vi "ARN Protokollkopf.vi"() -> (0 "Angehängtes Array":T1[][](array[typedef]), 3 "Kopfzeile":string[](array[string]))   [LabVIEW 2020, in "EPA 1065.lvlib" / "ARN Test 1065-305.lvlib"]
uses:
  ARN Test 1065-305.lvlib
  Visualisierungs Elemente/String - Ausgabefeld.ctl
  Seiten/FT-IR/FGV FT-IR Gasliste Aktionen.ctl
  Aktion FGV ARN Daten.ctl
  Sprachverwaltung/FGV Aktion Tabelle zerlegen.ctl
  Seiten/FT-IR/FT-IR.lvlib
  Sprachverwaltung/Sprachverwaltung.lvlib
  Seiten/System Einstellungen V2/System Einstellungen V2.lvlib
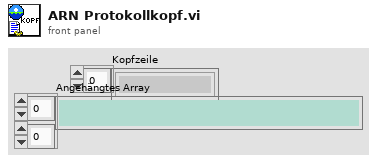
[diagram p1: front panel]
types:
  T1 = typedef "String - Ausgabefeld.ctl" = string
  T2 = typedef "Sprachverwaltung.lvlib/FGV Aktion Tabelle zerlegen.ctl" = enum16{"laden", "vereinzeln", "speichern"}
  T3 = typedef "FT-IR.lvlib/FGV FT-IR Gasliste Aktionen.ctl" = enum16{"lesen", "Gasliste FT-IR", "Gasliste ausgelesen", "laden", "speichern", "löschen"}
  T4 = typedef "EPA 1065.lvlib/ARN Test 1065-305.lvlib/Aktion FGV ARN Daten.ctl" = enum16{"Lesen", "laden", "speichern", "ARN Daten", "Rohdaten", "Rohdaten löschen", "Zeitstempel", "SNR Ergebnis"}
  T5 = typedef "EPA 1065.lvlib/ARN Test 1065-305.lvlib/Allgemeine Einstellungen.ctl" = cluster{"Bearbeiter:":string, "Analysator":T6, "Komponente:":u16, "Gasflaschen Nr.:":string, "Accuracy":dbl, "Sollwert":dbl, "Modus":T7, "Pfad:":path, "Textname:":string, "CG Aufschaltzeit:":dbl, "Einheit":string, "N2 Aufschaltzeit:":dbl, "Gasflasche":T8, "Konfig Gasflasche":T9}
  T6 = typedef "System Einstellungen V2.lvlib/Analysatoren.ctl" = string
  T7 = typedef "EPA 1065.lvlib/T90 Test 1065-308.lvlib/Modus.ctl" = u16
  T8 = typedef "System Einstellungen V2.lvlib/Gasflasche Auswahl.ctl" = u16
  T9 = typedef "System Einstellungen V2.lvlib/Konfig Gasflasche.ctl" = bool
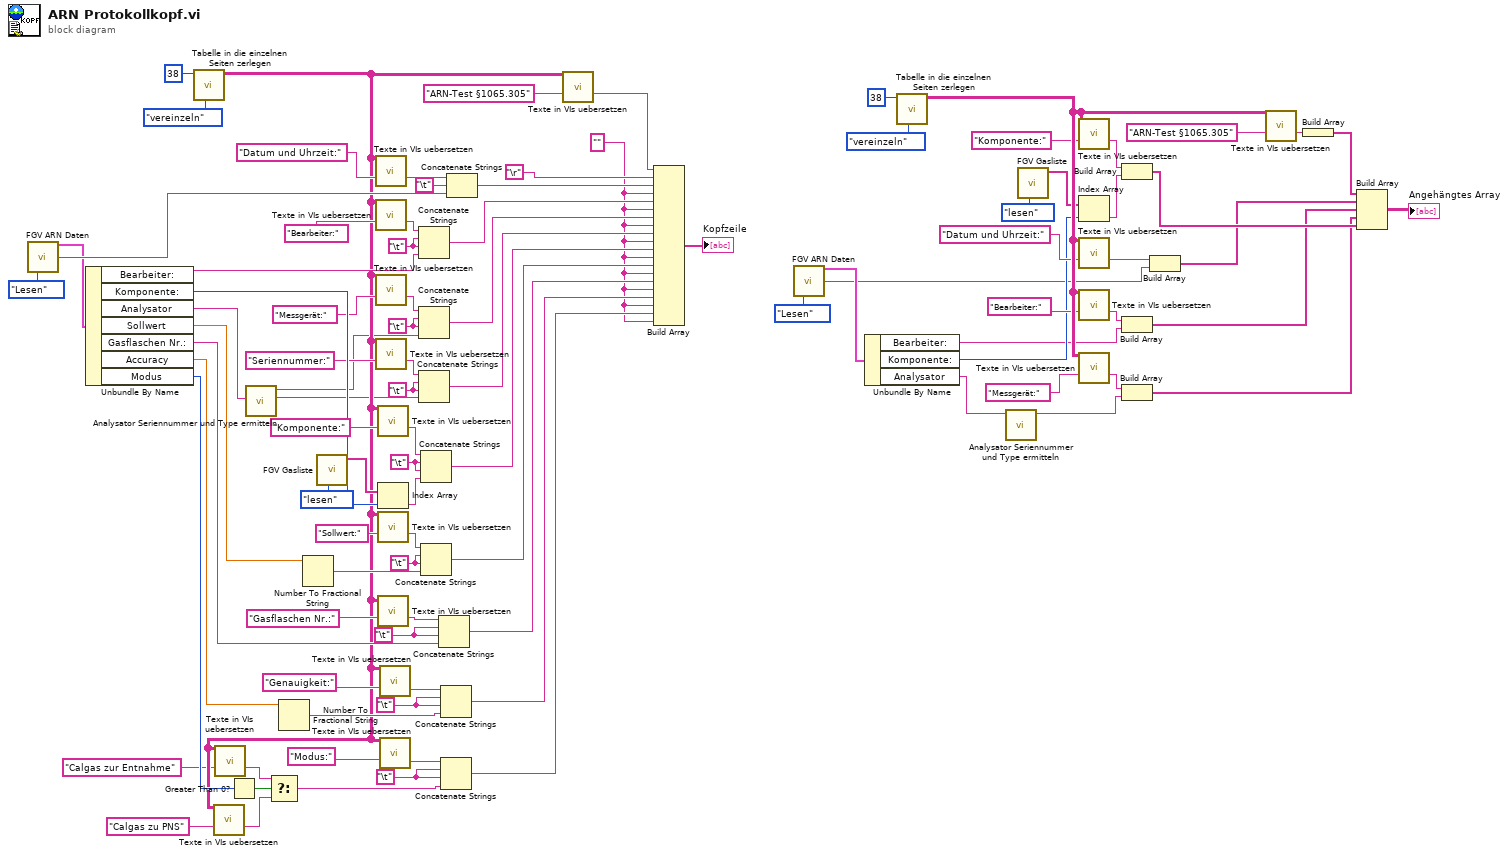
[diagram p0: block diagram]
diagram:
  w18 = "\t"
  w22 = "\t"
  w27 = "\t"
  w34 = "\t"
  w37 = "\t"
  w83 = "\t"
  w85 = "\t"
  w11 = "" ("Element")
  w92 = "\t"
  n1 = call "FGV ARN Daten.vi"("Aktion"=Aktion_FGV_ARN_Daten."Lesen") -> ("ARN Konfig Daten"=w90:T5, "Zeitstempel"=w91:string)  [unwired: 9 in, 4 out]
  n2 = Unbundle By Name(w90) -> ("Bearbeiter:"=w89:string, "Komponente:"=w86:u16, "Analysator"=w5:T6, "Sollwert"=w32:dbl, "Gasflaschen Nr.:"=w26:string, "Accuracy"=w19:dbl, "Modus"=w15:T7)
  n3 = call "Tabelle in die einzelnen Seiten zerlegen.vi"("Aktion"=FGV_Aktion_Tabelle_zerlegen."vereinzeln", "Index (Seite)"=38) -> ("Sprachliste"=w10:string[][])  [unwired: 7 in, 2 out]
  n4 = call "Texte in VIs uebersetzen.vi"("Sprachliste"=w10, "String zum Übersetzen"="Calgas zu PNS" ("f")) -> ("String zum Übersetzen"=w7:string)  [unwired: 9 in, 4 out]
  n5 = call "Texte in VIs uebersetzen.vi"("Sprachliste"=w10, "String zum Übersetzen"="Calgas zur Entnahme") -> ("String zum Übersetzen"=w6:string)  [unwired: 9 in, 4 out]
  n6 = Greater Than 0?(x=w15) -> (x > 0?=w14:bool)
  n7 = call "Analysator Seriennummer und Type ermitteln.vi"("Analysator"=w5) -> ("Type"=w2:string, "Name für Protokoll"=w1:string)  [unwired: 8 in, 1 out]
  n8 = Select(t=w6, s=w14, f=w7) -> (s? t:f=w13:string)
  n9 = Number To Fractional String(number=w19) -> (F-format string=w20:string)  [unwired: 3 in]
  n10 = Number To Fractional String(number=w32) -> (F-format string=w31:string)  [unwired: 3 in]
  n11 = call "FGV Gasliste.vi"("Aktionen"=FGV_FT-IR_Gasliste_Aktionen."lesen") -> ("Aktuelle Gasliste FT-IR"=w87:T1[])  [unwired: 8 in, 2 out]
  n12 = call "Texte in VIs uebersetzen.vi"("Sprachliste"=w10, "String zum Übersetzen"="Datum und Uhrzeit:") -> ("String zum Übersetzen"=w76:string)  [unwired: 9 in, 4 out]
  n13 = call "Texte in VIs uebersetzen.vi"("Sprachliste"=w10, "String zum Übersetzen"="Bearbeiter:") -> ("String zum Übersetzen"=w74:string)  [unwired: 9 in, 4 out]
  n14 = call "Texte in VIs uebersetzen.vi"("Sprachliste"=w10, "String zum Übersetzen"="Messgerät:") -> ("String zum Übersetzen"=w72:string)  [unwired: 9 in, 4 out]
  n15 = call "Texte in VIs uebersetzen.vi"("Sprachliste"=w10, "String zum Übersetzen"="Seriennummer:") -> ("String zum Übersetzen"=w39:string)  [unwired: 9 in, 4 out]
  n16 = call "Texte in VIs uebersetzen.vi"("Sprachliste"=w10, "String zum Übersetzen"="Komponente:") -> ("String zum Übersetzen"=w70:string)  [unwired: 9 in, 4 out]
  n17 = Index Array(array=w87, index=w86) -> (element=w82:T1)
  n18 = call "Texte in VIs uebersetzen.vi"("Sprachliste"=w10, "String zum Übersetzen"="Sollwert:") -> ("String zum Übersetzen"=w35:string)  [unwired: 9 in, 4 out]
  n19 = call "Texte in VIs uebersetzen.vi"("Sprachliste"=w10, "String zum Übersetzen"="Gasflaschen Nr.:") -> ("String zum Übersetzen"=w29:string)  [unwired: 9 in, 4 out]
  n20 = call "Texte in VIs uebersetzen.vi"("Sprachliste"=w10, "String zum Übersetzen"="Genauigkeit:") -> ("String zum Übersetzen"=w24:string)  [unwired: 9 in, 4 out]
  n21 = call "Texte in VIs uebersetzen.vi"("Sprachliste"=w10, "String zum Übersetzen"="Modus:") -> ("String zum Übersetzen"=w17:string)  [unwired: 9 in, 4 out]
  n22 = Concatenate Strings(w74, w92, w92, w89) -> (w41:string)
  n23 = Concatenate Strings(w72, w85, w85, w1) -> (w84:string)
  n24 = Concatenate Strings(w39, w37, w37, w2) -> (w36:string)
  n25 = Concatenate Strings(w70, w83, w83, w82) -> (w40:string)
  n26 = Concatenate Strings(w35, w34, w34, w31) -> (w30:string)
  n27 = Concatenate Strings(w29, w27, w27, w26) -> (w25:string)
  n28 = Concatenate Strings(w24, w22, w22, w20) -> (w21:string)
  n29 = Concatenate Strings(w17, w18, w18, w13) -> (w12:string)
  n30 = Concatenate Strings(w76, "\t", w91) -> (w93:string)
  n31 = call "Texte in VIs uebersetzen.vi"("Sprachliste"=w10, "String zum Übersetzen"="ARN-Test §1065.305") -> ("String zum Übersetzen"=w78:string)  [unwired: 9 in, 4 out]
  n32 = Build Array(w78, "\r", w93, w11, w41, w11, w84, w11, w36, w11, w40, w11, w30, w11, w25, w11, w21, w11, w12, w11) -> (→"Kopfzeile":string[])
  n33 = call "FGV ARN Daten.vi"("Aktion"=Aktion_FGV_ARN_Daten."Lesen") -> ("ARN Konfig Daten"=w48:T5, "Zeitstempel"=w46:string)  [unwired: 9 in, 4 out]
  n34 = Unbundle By Name(w48) -> ("Bearbeiter:"=w49:string, "Komponente:"=w52:u16, "Analysator"=w4:T6)
  n35 = call "Tabelle in die einzelnen Seiten zerlegen.vi"("Aktion"=FGV_Aktion_Tabelle_zerlegen."vereinzeln", "Index (Seite)"=38) -> ("Sprachliste"=w67:string[][])  [unwired: 7 in, 2 out]
  n36 = call "Analysator Seriennummer und Type ermitteln.vi"("Analysator"=w4) -> ("Name für Protokoll"=w3:string)  [unwired: 8 in, 2 out]
  n37 = call "FGV Gasliste.vi"("Aktionen"=FGV_FT-IR_Gasliste_Aktionen."lesen") -> ("Aktuelle Gasliste FT-IR"=w51:T1[])  [unwired: 8 in, 2 out]
  n38 = call "Texte in VIs uebersetzen.vi"("Sprachliste"=w67, "String zum Übersetzen"="Komponente:") -> ("String zum Übersetzen"=w66:string)  [unwired: 9 in, 4 out]
  n39 = Index Array(array=w51, index=w52) -> (element=w54:T1)
  n40 = call "Texte in VIs uebersetzen.vi"("Sprachliste"=w67, "String zum Übersetzen"="Datum und Uhrzeit:") -> ("String zum Übersetzen"=w60:string)  [unwired: 9 in, 4 out]
  n41 = call "Texte in VIs uebersetzen.vi"("Sprachliste"=w67, "String zum Übersetzen"="Bearbeiter:") -> ("String zum Übersetzen"=w62:string)  [unwired: 9 in, 4 out]
  n42 = call "Texte in VIs uebersetzen.vi"("Sprachliste"=w67, "String zum Übersetzen"="Messgerät:") -> ("String zum Übersetzen"=w64:string)  [unwired: 9 in, 4 out]
  n43 = Build Array(w66, w54) -> (w55:T1[])
  n44 = Build Array(w62, w49) -> (w47:string[])
  n45 = Build Array(w64, w3) -> (w53:string[])
  n46 = Build Array(w60, w46) -> (w44:string[])
  n47 = call "Texte in VIs uebersetzen.vi"("Sprachliste"=w67, "String zum Übersetzen"="ARN-Test §1065.305") -> ("String zum Übersetzen"=w58:string)  [unwired: 9 in, 4 out]
  n48 = Build Array(w58) -> (w43:string[])
  n49 = Build Array(w43, w44, w47, w53, w55) -> (→"Angehängtes Array":T1[][])
